vi "Error Handler.vi"(8 "error in (no error)":errorcluster, 11 "queue in":refnum<queue>) -> (0 "error out":errorcluster, 3 "queue out":refnum<queue>)   [LabVIEW 2018]
uses:
  Ctls/QueueData.ctl
  Ctls/State.ctl
  Ctls/CmdData.ctl
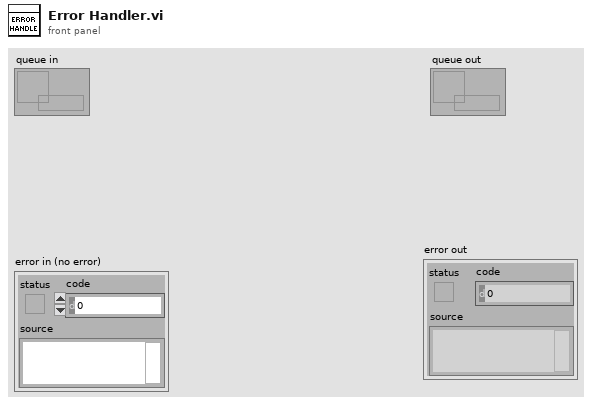
[diagram p1: front panel]
types:
  T1 = typedef "State.ctl" = enum16{"poll log data command", "poll control command", "display update", "init", "send bool command", "send float command", "datalog", "error", "fix rating rpm 1", "fix rating rpm 2", "fix both rating rpm", "fix rating rpm all", "terminate", "log Motor Speed Setting"}
  T2 = typedef "QueueData.ctl" = cluster{"State":T1, "Command Data":T3}
  T3 = typedef "CmdData.ctl" = cluster{"Address Areas":u8, "Data Block #":u16, "Start Address (bytes)":u32, "Write Data Float":sgl, "Bit #":u16, "Write Data Boolean":bool}
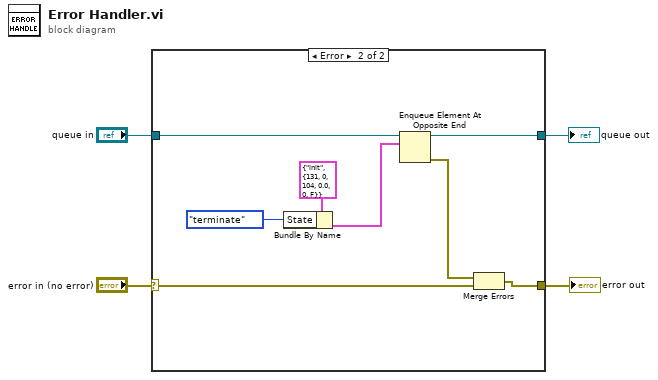
[diagram p0: block diagram]
diagram:
  n1 = case shown="Error" "error in (no error)" {
    selector: "error in (no error)" -> [w6 w8]
    tunnel: [w6 w7] -> w3
    tunnel: "queue in" -> [w5 w14]
    tunnel: [w5 w13] -> w1
    frame No Error {
    }
    frame Error {
      n2 = Bundle By Name(cluster=T2 {"State"=enum."init", "Command Data"={"Address Areas"=131, "Data Block #"=0, "Start Address (bytes)"=104, "Write Data Float"=0.0, "Bit #"=0, "Write Data Boolean"=FALSE}} ("QData"), "State"=State."terminate") -> (w11:T2)
      n3 = Enqueue Element At Opposite End(queue=w14, element=w11) -> (queue out=w13:refnum<queue>, error out=w9:errorcluster)  [unwired: 2 in, 1 out]
      n4 = Merge Errors(w9, w8) -> (w7:errorcluster)
    }
  }
  "error out" <- w3
  "queue out" <- w1
